vi "OA Get Number Of Pre Set Modes.vi"(8 "error in (no error)":errorcluster, 11 "puiNumberOfModes":u32) -> (0 "error out":errorcluster, 2 "function return":u32, 3 "puiNumberOfModes out":u32)   [LabVIEW 2014, in "atmcd32d.lvlib"]
doc: "unsigned int WINAPI OA_GetNumberOfPreSetModes(unsigned int * const puiNumberOfModes);"
uses:
  atmcd32d.lvlib
  atmcd32d.dll
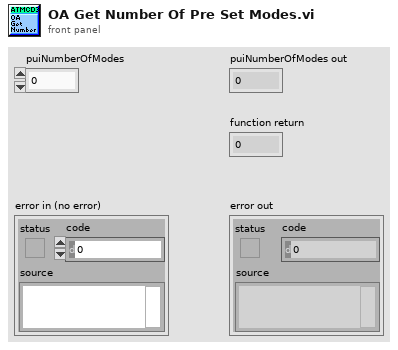
[diagram p1: front panel]
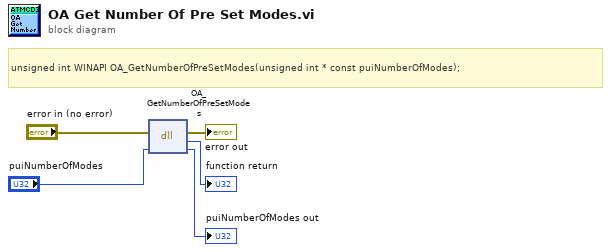
[diagram p0: block diagram]
diagram:
  # "unsigned int WINAPI OA_GetNumberOfPreSetModes(unsigned int * const puiNumberOfModes);"
  n1 = dll-call lib="C:/Users/Bakir/Documents/Lambda2-Testing/lib/Andorlib/atmcd32d.*" fn="OA_GetNumberOfPreSetModes"(error in="error in (no error)", "puiNumberOfModes"="puiNumberOfModes") -> (error out=→"error out":errorcluster, →"function return":u32, "puiNumberOfModes"=→"puiNumberOfModes out":u32)  [unwired: 2 in, 1 out]
